vi "Replace Value on Key Line.vi"(6 "key":string, 8 "error in (no error)":errorcluster, 9 "new value":string, 10 "prev value":string, 11 "line in":string) -> (0 "error out":errorcluster, 3 "line out":string)   [LabVIEW 2012, in "configlib.lvlib"]
uses:
  configlib.lvlib
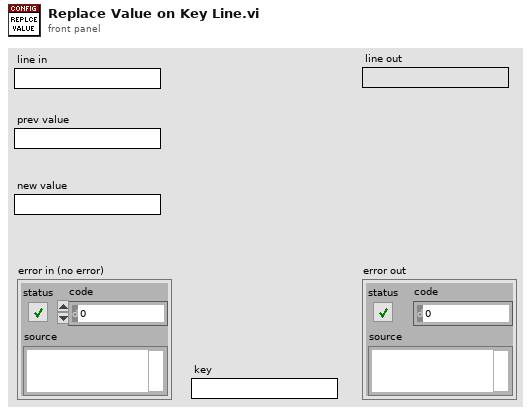
[diagram p1: front panel]
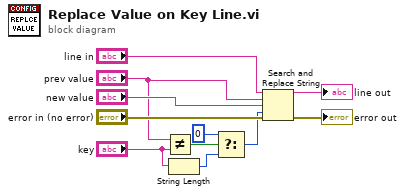
[diagram p0: block diagram]
diagram:
  n1 = Not Equal?(x="prev value", y="key") -> (x != y?=w8:bool)
  n2 = String Length(string="key") -> (length=w5:i32)
  n3 = Select(t=0, s=w8, f=w5) -> (s? t:f=w4:i32)
  n4 = Search and Replace String(input string="line in", search string="prev value", replace string="new value", offset=w4, error in="error in (no error)") -> (result string=→"line out":string, error out=→"error out":errorcluster)  [unwired: 3 in, 2 out]
